vi "BuildErrorFromCode_SG.vi"(8 "error in (no error)":errorcluster, 10 "Location":string, 11 "Error Code":u32) -> (0 "error out":errorcluster)   [LabVIEW 2012, in "SG-Lock.lvlib"]
uses:
  SG-Lock.lvlib
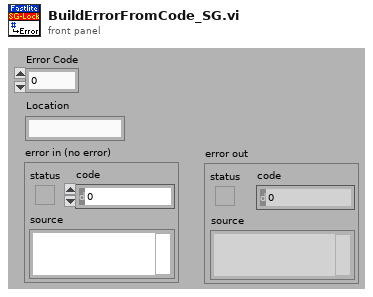
[diagram p1: front panel]
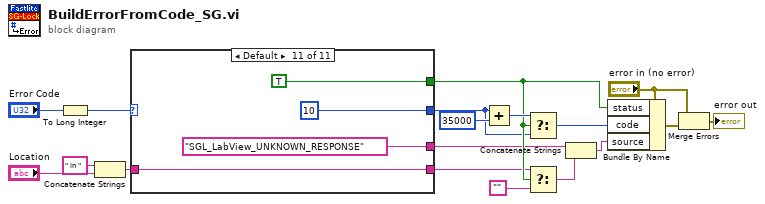
[diagram p0: block diagram]
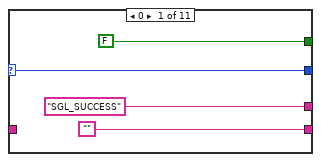
[diagram p2: hidden frame]
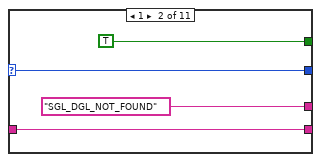
[diagram p3: hidden frame]
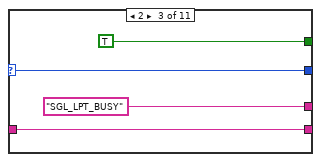
[diagram p4: hidden frame]
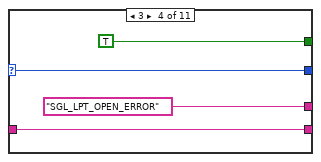
[diagram p5: hidden frame]
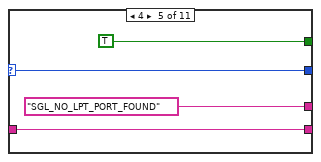
[diagram p6: hidden frame]
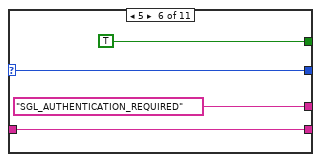
[diagram p7: hidden frame]
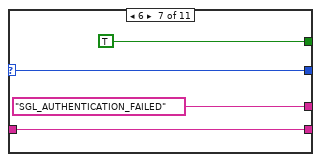
[diagram p8: hidden frame]
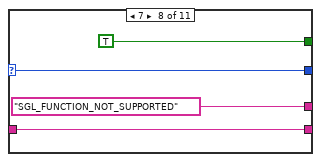
[diagram p9: hidden frame]
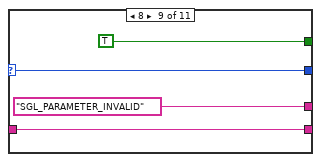
[diagram p10: hidden frame]
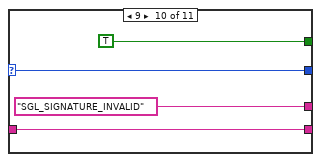
[diagram p11: hidden frame]
diagram:
  n1 = To Long Integer(number="Error Code") -> (32bit integer=w13:i32)
  n2 = Concatenate Strings(" in " ("string"), "Location") -> (w8:string)
  n3 = case shown="Default" w13 {
    selector: w13 -> [w20 w24 w28 w32 w36 w40 w44 w48 w52 w56 _]
    tunnel: ["SGL_SUCCESS" "SGL_DGL_NOT_FOUND" "SGL_LPT_BUSY" "SGL_LPT_OPEN_ERROR" "SGL_NO_LPT_PORT_FOUND" "SGL_AUTHENTICATION_REQUIRED" "SGL_AUTHENTICATION_FAILED" "SGL_FUNCTION_NOT_SUPPORTED" "SGL_PARAMETER_INVALID" "SGL_SIGNATURE_INVALID" "SGL_LabView_UNKNOWN_RESPONSE"] -> w2
    tunnel: [FALSE TRUE TRUE TRUE TRUE TRUE TRUE TRUE TRUE TRUE TRUE] -> w7
    tunnel: [w20 w24 w28 w32 w36 w40 w44 w48 w52 w56 u8 10] -> w1
    tunnel: ["" w23 w27 w31 w35 w39 w43 w47 w51 w55 w59] -> w6
    tunnel: w8 -> [_ w23 w27 w31 w35 w39 w43 w47 w51 w55 w59]
    frame 0 {
    }
    frame 1 {
    }
    frame 2 {
    }
    frame 3 {
    }
    frame 4 {
    }
    frame 5 {
    }
    frame 6 {
    }
    frame 7 {
    }
    frame 8 {
    }
    frame 9 {
    }
    frame Default {
    }
  }
  n4 = Add(x=w1, y=35000) -> (x+y=w14:i32)
  n5 = Select(t=w14, s=w7, f=w1) -> (s? t:f=w12:i32)
  n6 = Select(t=w6, s=w7, f="") -> (s? t:f=w4:string)
  n7 = Concatenate Strings(w2, w4) -> (w3:string)
  n8 = Bundle By Name(cluster="error in (no error)", "status"=w7, "code"=w12, "source"=w3) -> (w16:errorcluster)
  n9 = Merge Errors("error in (no error)", w16) -> (→"error out":errorcluster)
